vi "base format to strings.vi"(8 "error in":errorcluster, 11 "format":T4) -> (0 "error out":errorcluster, 3 "data":T1)   [LabVIEW 2013, in "NISE_CEF_TreeSerializer.lvlib"]
uses:
  NISE_CEF_TreeSerializer.lvlib
  base file format.ctl
  file data format.ctl
  hierarchy element.ctl
  instance data.ctl
  serializable configuration/NISE_CEF_serializable configuration.lvclass
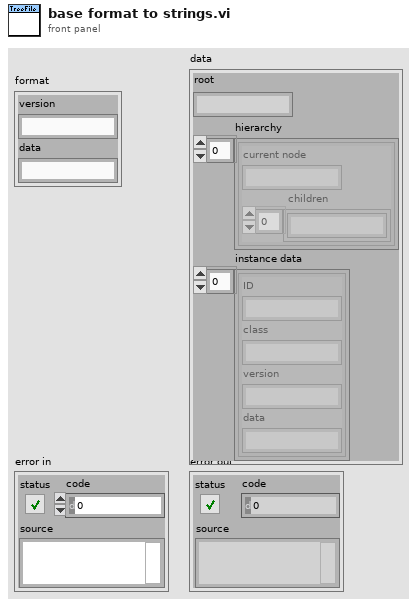
[diagram p1: front panel]
types:
  T1 = typedef "NISE_CEF_TreeSerializer.lvlib/file data format.ctl" = cluster{"root":string, "hierarchy":T2[], "instance data":T3[]}
  T2 = typedef "NISE_CEF_TreeSerializer.lvlib/hierarchy element.ctl" = cluster{"current node":string, "children":string[]}
  T3 = typedef "NISE_CEF_TreeSerializer.lvlib/instance data.ctl" = cluster{"ID":string, "class":string, "version":string, "data":string}
  T4 = typedef "NISE_CEF_TreeSerializer.lvlib/base file format.ctl" = cluster{"version":string, "data":string}
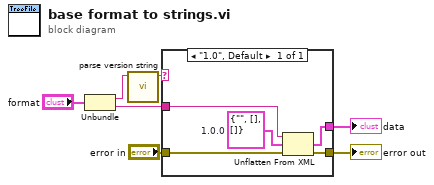
[diagram p0: block diagram]
diagram:
  n1 = Unbundle("format") -> ("version"=w6:string, "data"=w4:string)
  n2 = call "parse version string.vi"("full version"=w6) -> ("major.minor version"=w5:string)  [unwired: 7 in, 3 out]
  n3 = case shown="\"1.0\", Default" w5 {
    tunnel: w4 -> [w12]
    tunnel: [w10] -> w3
    tunnel: "error in" -> [w9]
    tunnel: [w8] -> w1
    frame "1.0", Default {
      w11 = T1 {"root"="", "hierarchy"=[], "instance data"=[]}  # 1.0.0
      n4 = Unflatten From XML(xml string=w12, type=w11, error in (no error)=w9) -> (value=w8:T1, error out=w10:errorcluster)
    }
  }
  "error out" <- w3
  "data" <- w1
